vi "Write Byte Count.vi"(8 "error in (no error)":errorcluster, 10 "Byte Count":u32 step=1 format="%.0g", 11 "ReadCommand in":refnum<class "ReadCommand.lvclass">) -> (0 "error out":errorcluster, 3 "ReadCommand out":refnum<class "ReadCommand.lvclass">)   [LabVIEW 2023, in "HAF.lvlib" / "ReadCommand.lvclass"]
doc: "Sets a new Byte Count value."
uses:
  ReadCommand.lvclass
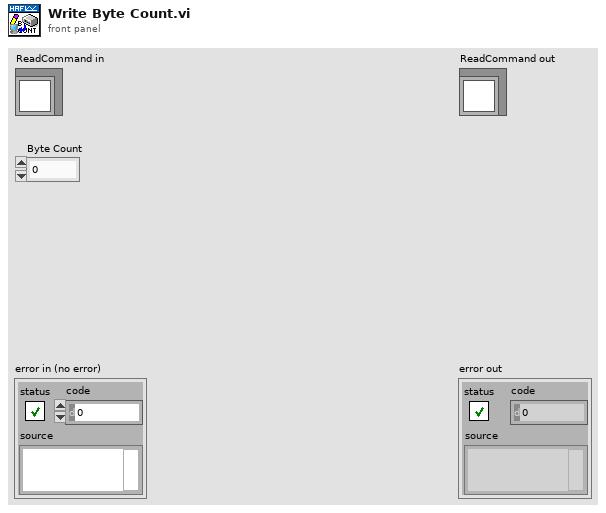
[diagram p1: front panel]
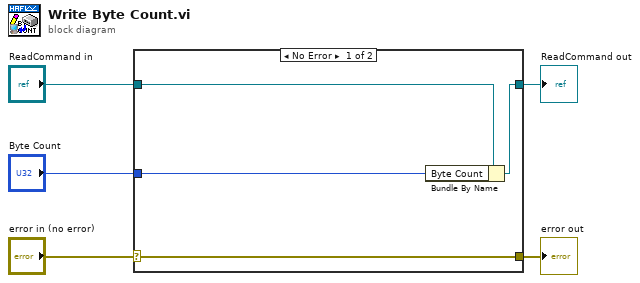
[diagram p0: block diagram]
diagram:
  n1 = case shown="No Error" "error in (no error)" {
    selector: "error in (no error)" -> [w9 w10]
    tunnel: [w9 w10] -> w4
    tunnel: [w7 w11] -> w2
    tunnel: "ReadCommand in" -> [w8 w11]
    tunnel: "Byte Count" -> [w6 _]
    frame No Error {
      n2 = Bundle By Name(cluster=w8, "Byte Count"=w6) -> (w7:refnum<class "ReadCommand.lvclass">)
    }
    frame Error {
    }
  }
  "error out" <- w4
  "ReadCommand out" <- w2
